vi "PH_DIM.add Double Array Service.vi"(0 "i ref in":refnum<vi>, 1 "Service Name":string="N/A", 2 "Double Value Array":dbl[](array[numeric]), 5 "error in (no error)":errorcluster) -> (14 "i ref out":refnum<vi>, 17 "Service ID":i32, 19 "error out":errorcluster)   [LabVIEW 2014, in "PH_Common.lvlib"]
doc: "This VI publishes a double number array opening a service \"<instancename>ServiceName\", if no error comes in, and the ServiceName is not N/A. For further use, the Service ID is given out (it is \"-1\" if the service has not been added)."
uses:
  PH_Common.lvlib
  lib.lib/DimLVEvent/LVDimInterface/LVDimInterface.lvlib
  CSCore/CSSystem/CSSystemLib/CSSystemLib.lvlib
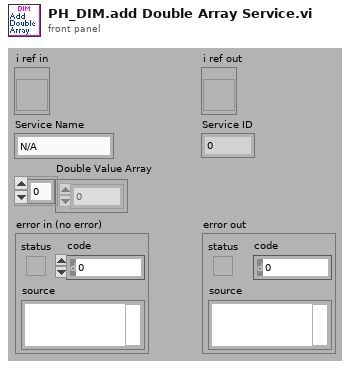
[diagram p1: front panel]
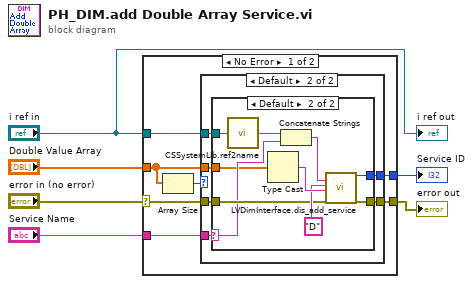
[diagram p0: block diagram]
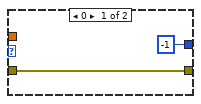
[diagram p2: hidden frame]
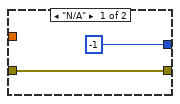
[diagram p3: hidden frame]
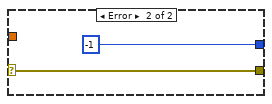
[diagram p4: hidden frame]
diagram:
  n1 = case shown="No Error" "error in (no error)" {
    selector: "error in (no error)" -> [w10 w35]
    tunnel: [w13 -1 ("my_serviceID")] -> w6
    tunnel: [w12 w35] -> w5
    tunnel: "Double Value Array" -> [w8 _]
    tunnel: "i ref in" -> [w11 _]
    tunnel: "Service Name" -> [w9 _]
    frame No Error {
      n2 = Array Size(array=w8) -> (size(s)=w7:i32)
      n3 = case shown="Default" w7 {
        tunnel: [-1 ("my_serviceID") w21] -> w13
        tunnel: [w15 w20] -> w12
        tunnel: w11 -> [_ w19]
        tunnel: w10 -> [w15 w18]
        tunnel: w9 -> [_ w17]
        tunnel: w8 -> [_ w16]
        frame 0 {
        }
        frame Default {
          n4 = case shown="Default" w17 {
            selector: w17 -> [_ w26]
            tunnel: [-1 ("my_serviceID") w25] -> w21
            tunnel: [w23 w27] -> w20
            tunnel: w19 -> [_ w29]
            tunnel: w18 -> [w23 w28]
            tunnel: w16 -> [_ w24]
            frame "N/A" {
            }
            frame Default {
              n5 = call "CSSystemLib.ref2name.vi"("obj refnum"=w29) -> ("name"=w31:string)
              n6 = Type Cast(x=w24) -> (*(type *) &x=w33:string)  [unwired: 1 in]
              n7 = Concatenate Strings(w31, w26) -> (w30:string)
              n8 = call "LVDimInterface.dis_add_service.vi"("serviceName"=w30, "typeDescriptor"="D", "data"=w33, "error in (no error)"=w28) -> ("my_serviceID"=w25:i32, "error out"=w27:errorcluster)  [unwired: 14 in]
            }
          }
        }
      }
    }
    frame Error {
    }
  }
  "Service ID" <- w6
  "error out" <- w5
  "i ref out" <- "i ref in"
